vi "realscan (SubVI).vi"(11 "stop":bool) -> (1 "enviroment":u32[][](graph), 2 "Array":u32[][](array[colorbox]), 3 "new picture":picture)   [LabVIEW 2011]
panel:
  in  "dimension size 2":i32=51
  in  "dimension size":i32=51
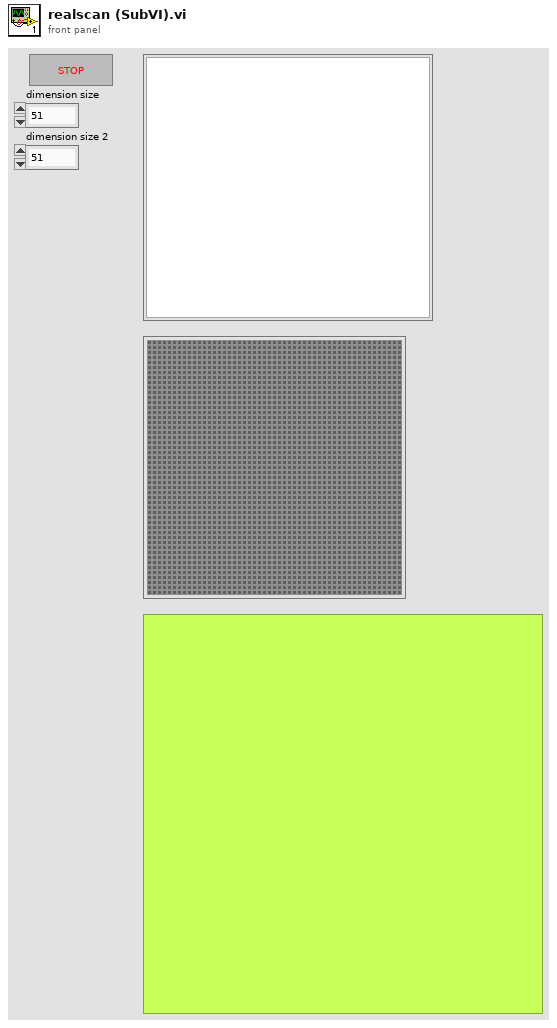
[diagram p1: front panel]
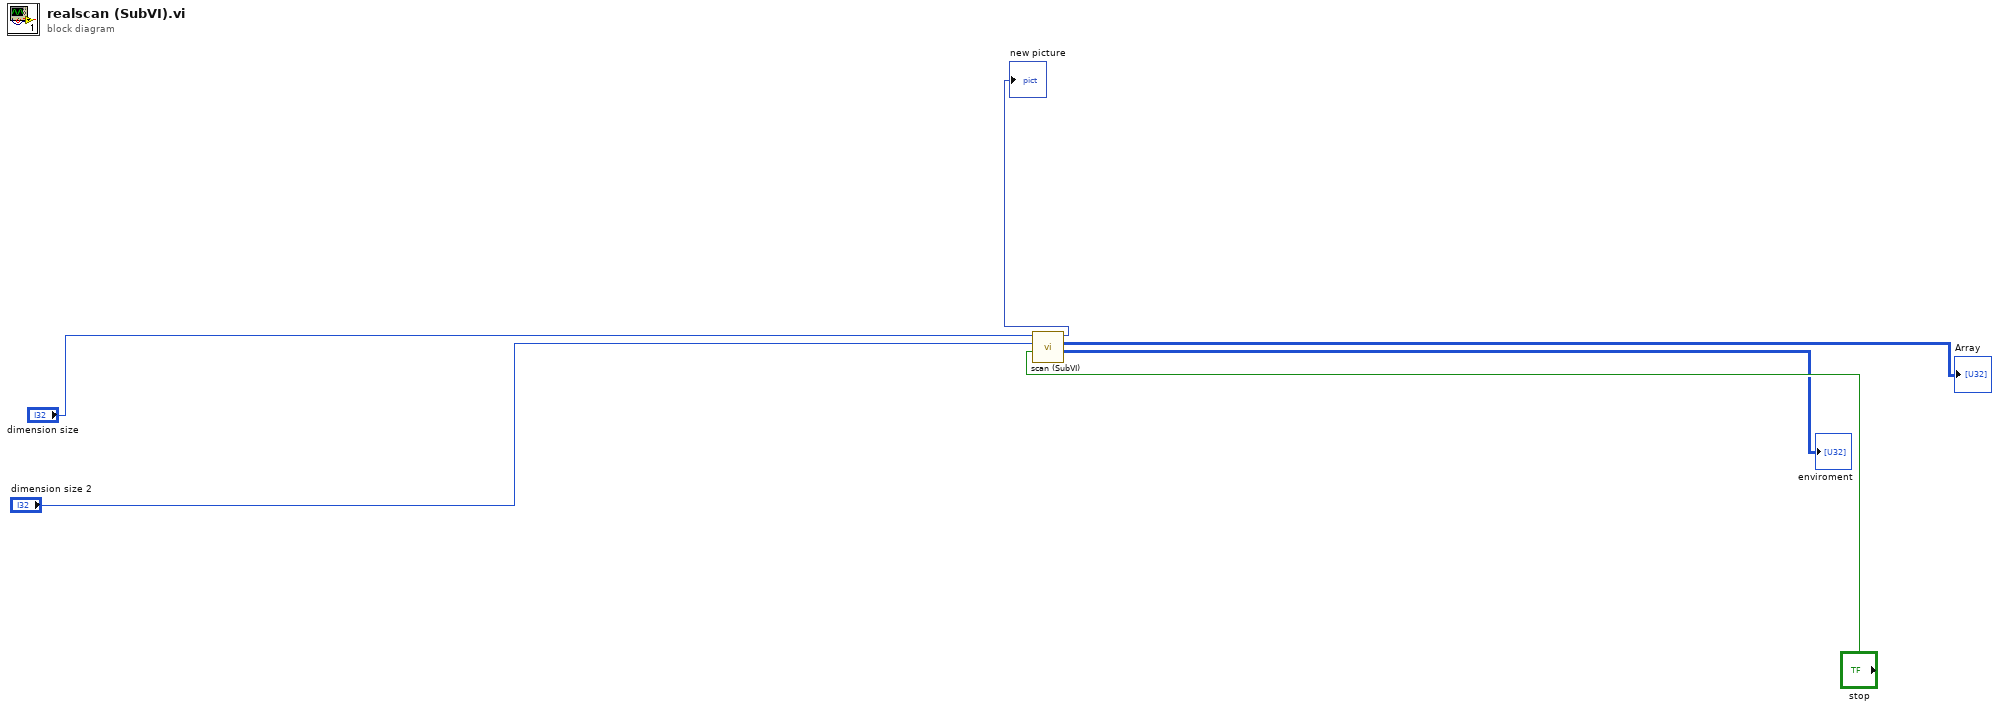
[diagram p0: block diagram]
diagram:
  n1 = call "scan (SubVI).vi"("stop"="stop", "dimension size 2"="dimension size 2", "dimension size"="dimension size") -> ("enviroment"=→"enviroment":u32[][], "Array"=→"Array":u32[][], "new picture"=→"new picture":picture)  [unwired: 6 in]
